vi "读取数值.vi"(8 "error in (no error)":errorcluster, 10 "Slave ID":u8=1, 11 "MB session in":refnum<class "MB_Master.lvclass">) -> (0 "error out":errorcluster, 2 "读取值":cluster{"瞬时流量":sgl, "累计流量":sgl, "水位":sgl}, 3 "MB session out":refnum<class "MB_Master.lvclass">)   [LabVIEW 2016, in "WL-1A1.lvlib"]
uses:
  WL-1A1.lvlib
  <vilib>/Plasmionique/MB Master/MB_Master/MB_Master.lvclass
  <vilib>/Plasmionique/MB Master/MB Master.lvlib
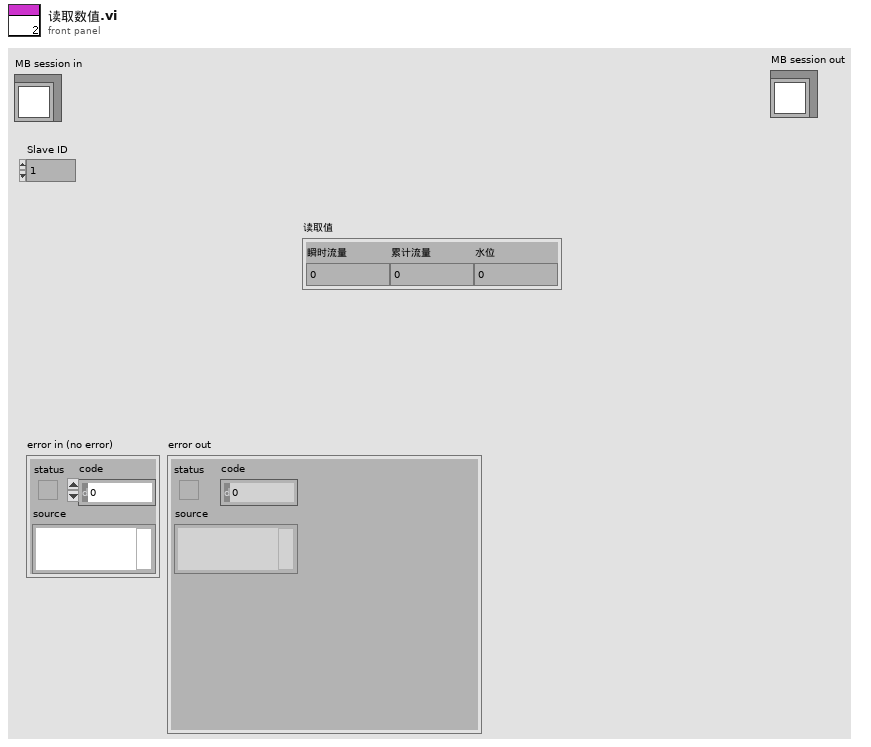
[diagram p1: front panel]
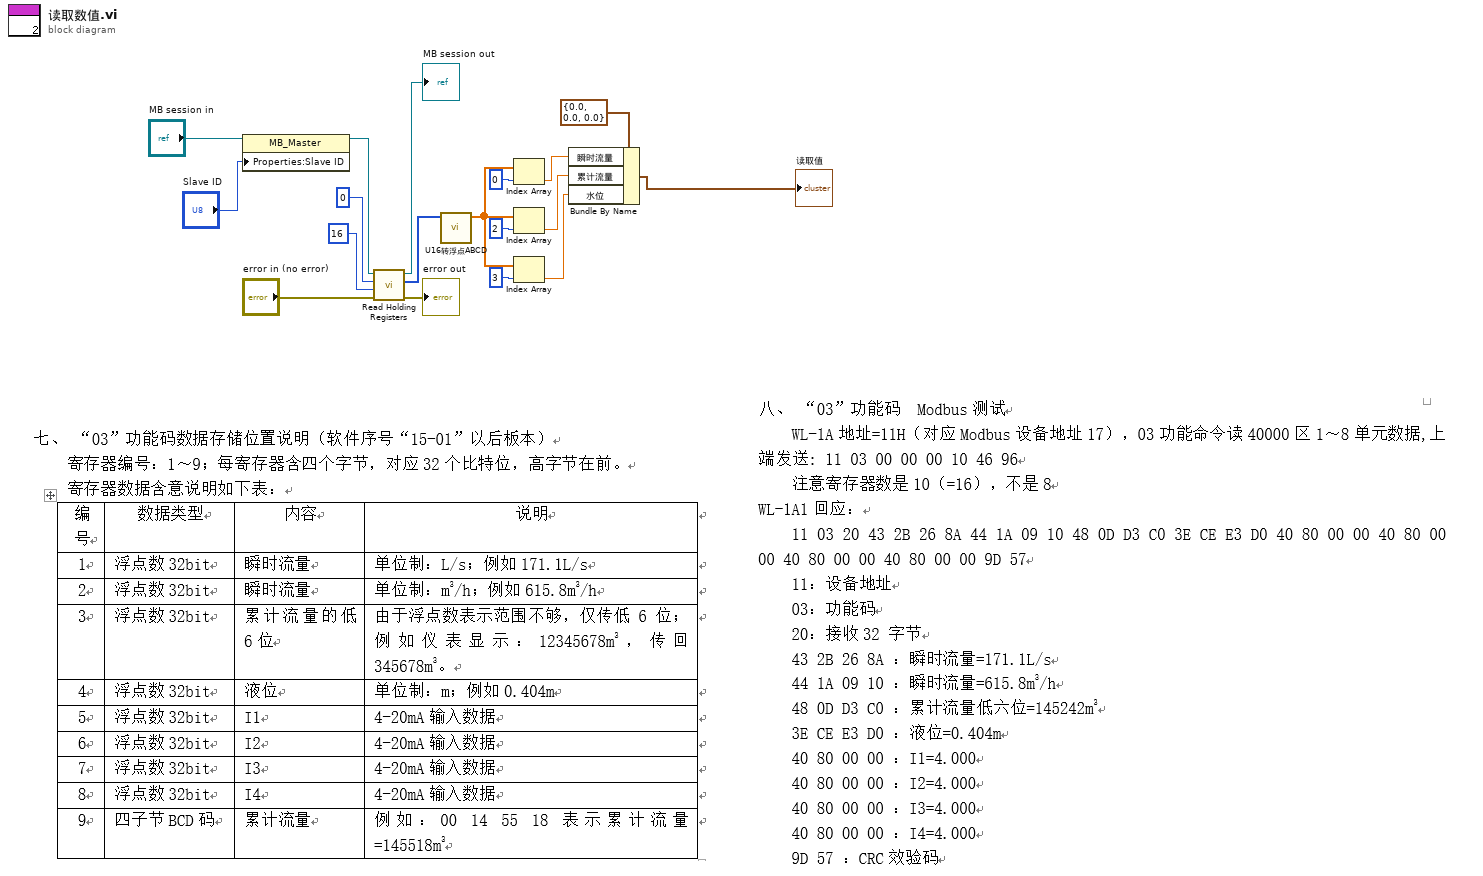
[diagram p0: block diagram]
diagram:
  n1 = property class="MB_Master"(reference="MB session in", "Properties:Slave ID"="Slave ID") -> (reference out=w16:refnum<class "MB_Master.lvclass">)  [unwired: 1 in, 1 out]
  n2 = call <vilib>:"Read Holding Registers.vi"("error in (no error)"="error in (no error)", "quantity"=u16 16, "starting address"=u16 0, "MB session in"=w16) -> ("error out"=→"error out":errorcluster, "Registers"=w10:u16[], "MB session out"=→"MB session out":refnum<class "MB_Master.lvclass">)  [unwired: 5 in]
  n3 = call "U16转浮点ABCD.vi"("U16"=w10) -> ("Float ABCD"=w4:sgl[])  [unwired: 10 in]
  n4 = Index Array(array=w4, index=0 ("索引")) -> (element=w8:sgl)
  n5 = Index Array(array=w4, index=2 ("索引")) -> (element=w7:sgl)
  n6 = Index Array(array=w4, index=3 ("索引")) -> (element=w5:sgl)
  n7 = Bundle By Name(cluster=cluster{"瞬时流量":sgl, "累计流量":sgl, "水位":sgl} {"瞬时流量"=0.0, "累计流量"=0.0, "水位"=0.0} ("读取值"), "瞬时流量"=w8, "累计流量"=w7, "水位"=w5) -> (→"读取值":cluster{"瞬时流量":sgl, "累计流量":sgl, "水位":sgl})
